vi "测试类型1自动测试一组.vi"() -> ()   [LabVIEW 2010]
uses:
  全局量/试验配置信息.vi
panel:
  in  "测试值":dbl[](array[numeric])
  out "EVENT_KEY":string
  out "bRece":bool
  out "bSend":bool
  out "第几个":i32
  out "bStop":bool
  out "数据组数":i32
  out "第几组":i32
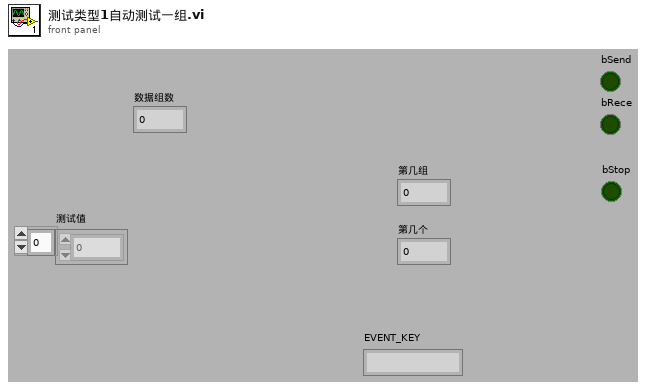
[diagram p1: front panel]
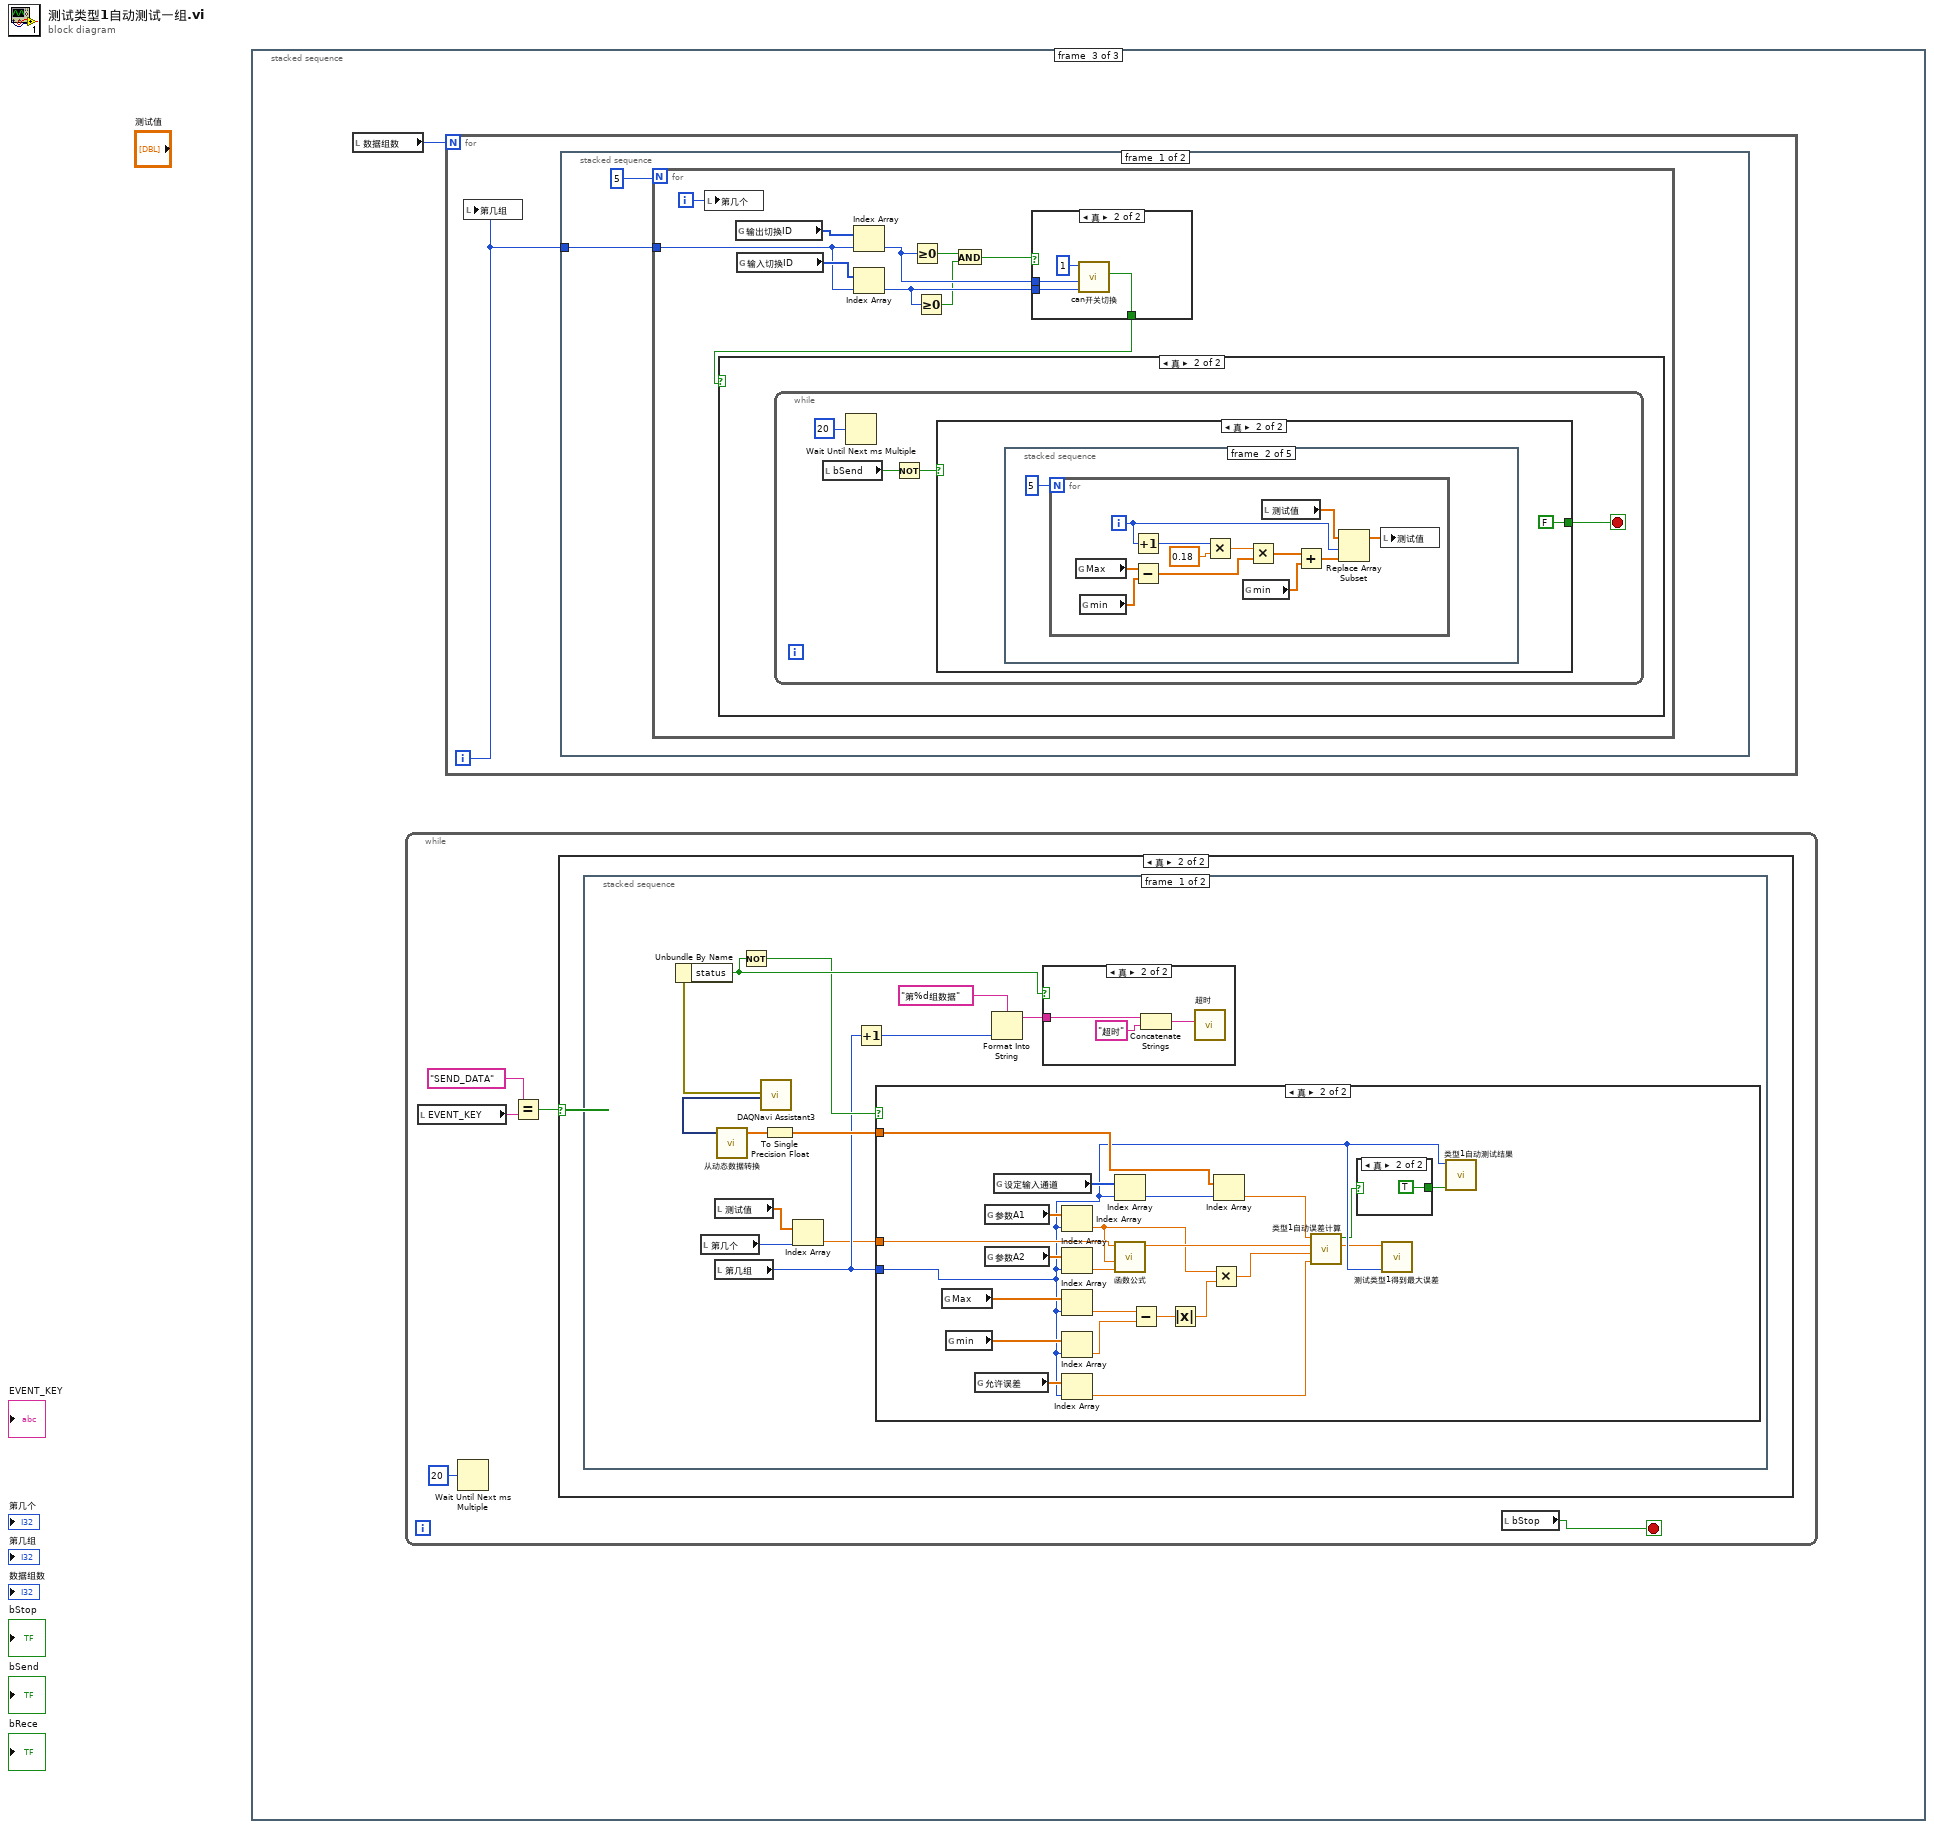
[diagram p0: block diagram]
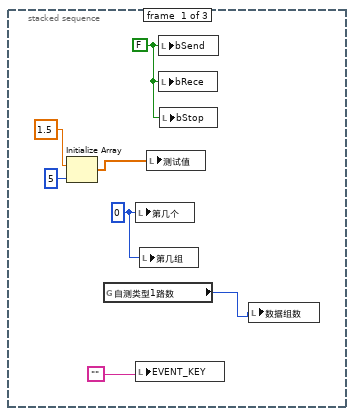
[diagram p2: hidden frame]
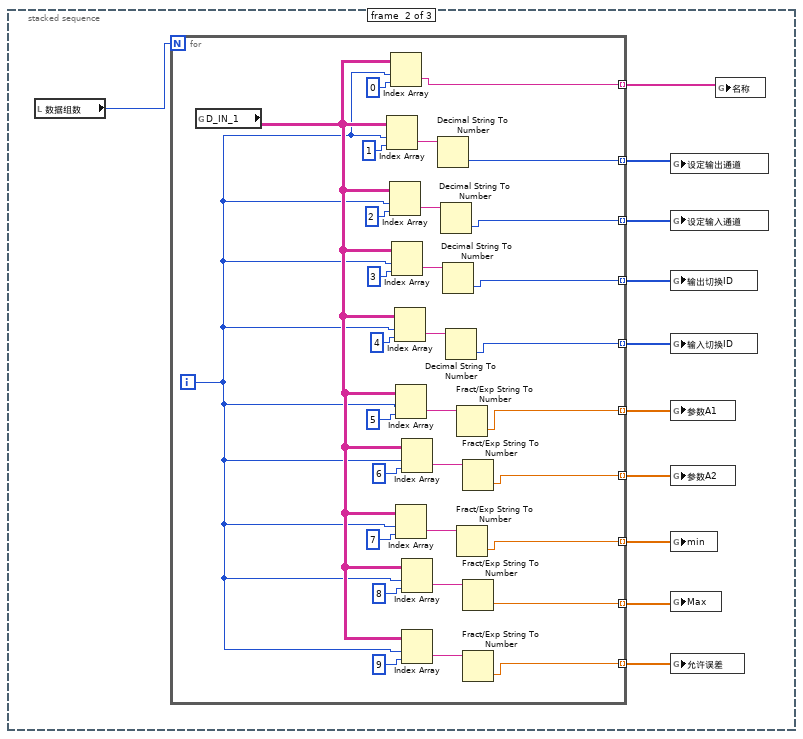
[diagram p3: hidden frame]
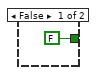
[diagram p7: hidden frame]
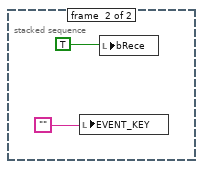
[diagram p8: hidden frame]
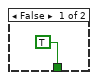
[diagram p9: hidden frame]
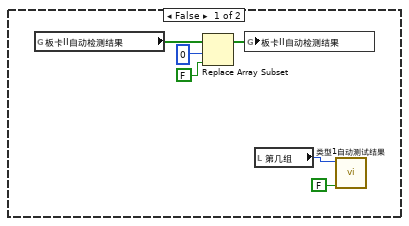
[diagram p10: hidden frame]
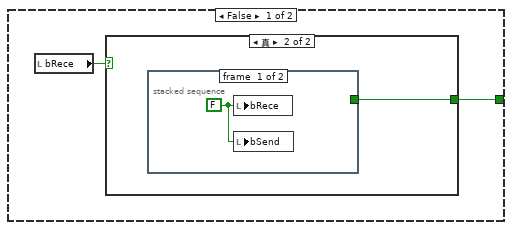
[diagram p11: hidden frame]
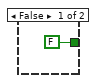
[diagram p12: hidden frame]
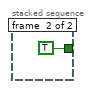
[diagram p13: hidden frame]
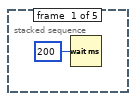
[diagram p14: hidden frame]
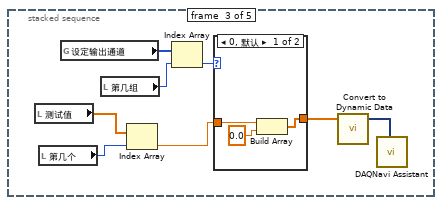
[diagram p15: hidden frame]
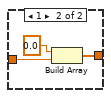
[diagram p16: hidden frame]
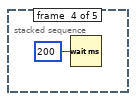
[diagram p17: hidden frame]
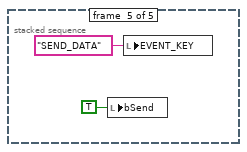
[diagram p18: hidden frame]
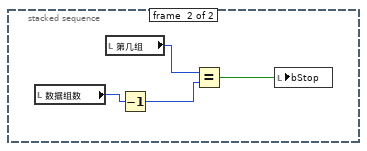
[diagram p19: hidden frame]
diagram:
  n1 = stacked-sequence {
    frame #0 {
      w6 = FALSE
      w7 = 0 ("同步A")
      n2 = Initialize Array(1.5 ("数值"), 5 ("维数大小")) -> (w2:dbl[])
      n3 = global read "试验配置信息.vi" "自测类型1路数"() -> (w1:i32)
      n4 = local write "第几个"(w7) -> ()
      n5 = local write "EVENT_KEY"("") -> ()
      n6 = local write "第几组"(w7) -> ()
      n7 = local write "测试值"(w2) -> ()
      n8 = local write "bSend"(w6) -> ()
      n9 = local write "bRece"(w6) -> ()
      n10 = local write "bStop"(w6) -> ()
      n11 = local write "数据组数"(w1) -> ()
    }
    frame #1 {
      n12 = local read "数据组数"() -> (w9:i32)
      n13 = for {
        N: w9 -> [_]
        tunnel: [w31] -> w10 mode=indexing
        tunnel: [w30] -> w11 mode=indexing
        tunnel: [w29] -> w12 mode=indexing
        tunnel: [w28] -> w13 mode=indexing
        tunnel: [w27] -> w14 mode=indexing
        tunnel: [w26] -> w15 mode=indexing
        tunnel: [w25] -> w16 mode=indexing
        tunnel: [w24] -> w17 mode=indexing
        tunnel: [w23] -> w18 mode=indexing
        tunnel: [w20] -> w8 mode=indexing
        i -> [w19]
        n14 = global read "试验配置信息.vi" "D_IN_1"() -> (w21:string[][])
        n15 = Index Array(array=w21, index (row)=w19, index (col)=1 ("禁用的索引 (列)")) -> (element=w49:string)
        n16 = Index Array(array=w21, index (row)=w19, index (col)=2 ("禁用的索引 (列)")) -> (element=w46:string)
        n17 = Index Array(array=w21, index (row)=w19, index (col)=0 ("禁用的索引 (列)")) -> (element=w20:string)
        n18 = Index Array(array=w21, index (row)=w19, index (col)=3 ("禁用的索引 (列)")) -> (element=w42:string)
        n19 = Index Array(array=w21, index (row)=w19, index (col)=4 ("禁用的索引 (列)")) -> (element=w45:string)
        n20 = Index Array(array=w21, index (row)=w19, index (col)=5 ("禁用的索引 (列)")) -> (element=w40:string)
        n21 = Index Array(array=w21, index (row)=w19, index (col)=7 ("禁用的索引 (列)")) -> (element=w35:string)
        n22 = Index Array(array=w21, index (row)=w19, index (col)=6 ("禁用的索引 (列)")) -> (element=w39:string)
        n23 = Index Array(array=w21, index (row)=w19, index (col)=8 ("禁用的索引 (列)")) -> (element=w36:string)
        n24 = Index Array(array=w21, index (row)=w19, index (col)=9 ("禁用的索引 (列)")) -> (element=w33:string)
        n25 = Decimal String To Number(string=w49) -> (number=w31:i32)  [unwired: 2 in, 1 out]
        n26 = Decimal String To Number(string=w46) -> (number=w30:i32)  [unwired: 2 in, 1 out]
        n27 = Decimal String To Number(string=w42) -> (number=w29:i32)  [unwired: 2 in, 1 out]
        n28 = Decimal String To Number(string=w45) -> (number=w28:i32)  [unwired: 2 in, 1 out]
        n29 = Fract/Exp String To Number(string=w40) -> (number=w27:dbl)  [unwired: 3 in, 1 out]
        n30 = Fract/Exp String To Number(string=w35) -> (number=w25:dbl)  [unwired: 3 in, 1 out]
        n31 = Fract/Exp String To Number(string=w39) -> (number=w26:dbl)  [unwired: 3 in, 1 out]
        n32 = Fract/Exp String To Number(string=w36) -> (number=w24:dbl)  [unwired: 3 in, 1 out]
        n33 = Fract/Exp String To Number(string=w33) -> (number=w23:dbl)  [unwired: 3 in, 1 out]
      }
      n34 = global write "试验配置信息.vi" "设定输出通道"(w10) -> ()
      n35 = global write "试验配置信息.vi" "设定输入通道"(w11) -> ()
      n36 = global write "试验配置信息.vi" "输出切换ID"(w12) -> ()
      n37 = global write "试验配置信息.vi" "输入切换ID"(w13) -> ()
      n38 = global write "试验配置信息.vi" "参数A1"(w14) -> ()
      n39 = global write "试验配置信息.vi" "参数A2"(w15) -> ()
      n40 = global write "试验配置信息.vi" "min"(w16) -> ()
      n41 = global write "试验配置信息.vi" "Max"(w17) -> ()
      n42 = global write "试验配置信息.vi" "允许误差"(w18) -> ()
      n43 = global write "试验配置信息.vi" "名称"(w8) -> ()
    }
    frame #2 {
      n44 = local read "数据组数"() -> (w50:i32)
      n45 = while {
        stop <- w51 stop-if-true
        n46 = local read "EVENT_KEY"() -> (w54:string)
        n47 = Wait Until Next ms Multiple(millisecond multiple=u32 20 ("毫秒倍数")) -> ()  [unwired: 1 out]
        n48 = Equal?(x="SEND_DATA" ("EVENT_KEY"), y=w54) -> (x = y?=w53:bool)
        n49 = case shown="真" w53 {
          frame False {
          }
          frame True {
            n50 = stacked-sequence {
              frame #0 {
                n51 = local read "第几个"() -> (w57:i32)
                n52 = local read "测试值"() -> (w58:dbl[])
                n53 = local read "第几组"() -> (w59:i32)
                n54 = call "DAQNavi Assistant3"() -> ("error out"=w64:errorcluster, "data out(DDT)"=w65:dynamicdata)  [unwired: 2 in, 16 out]
                n55 = Unbundle By Name(w64) -> ("status"=w68:bool)
                n56 = call "从动态数据转换"("Dynamic Data Type"=w65) -> ("Array"=w66:dbl[])  [unwired: 3 in]
                n57 = Not(x=w68) -> (.not. x?=w63:bool)
                n58 = To Single Precision Float(number=w66) -> (single precision float=w67:sgl[])
                n59 = Index Array(array=w58, index=w57) -> (element=w56:dbl)
                n60 = Increment(x=w59) -> (x+1=w62:i32)
                n61 = case shown="真" w63 {
                  tunnel: w67 -> [_ w92]
                  tunnel: w59 -> [_ w81]
                  tunnel: w56 -> [_ w82]
                  frame False {
                  }
                  frame True {
                    n62 = global read "试验配置信息.vi" "Max"() -> (w88:dbl[])
                    n63 = global read "试验配置信息.vi" "min"() -> (w89:dbl[])
                    n64 = global read "试验配置信息.vi" "允许误差"() -> (w87:dbl[])
                    n65 = global read "试验配置信息.vi" "参数A1"() -> (w91:dbl[])
                    n66 = global read "试验配置信息.vi" "参数A2"() -> (w90:dbl[])
                    n67 = global read "试验配置信息.vi" "设定输入通道"() -> (w94:u32[])
                    n68 = Index Array(array=w91, index=w81) -> (element=w74:dbl)
                    n69 = Index Array(array=w90, index=w81) -> (element=w75:dbl)
                    n70 = Index Array(array=w88, index=w81) -> (element=w85:dbl)
                    n71 = Index Array(array=w89, index=w81) -> (element=w84:dbl)
                    n72 = Index Array(array=w87, index=w81) -> (element=w78:dbl)
                    n73 = Index Array(array=w94, index=w81) -> (element=w93:u32)
                    n74 = call "函数公式.vi"("参数 b"=w75, "参数 a"=w74, "设定值 1"=w82) -> ("y"=w79:dbl)  [unwired: 5 in, 1 out]
                    n75 = Subtract(x=w85, y=w84) -> (x-y=w86:dbl)
                    n76 = Absolute Value(x=w86) -> (abs(x)=w73:dbl)
                    n77 = Multiply(x=w74, y=w73) -> (x*y=w72:dbl)
                    n78 = Index Array(array=w92, index=w93) -> (element=w80:sgl)
                    n79 = call "类型1自动误差计算.vi"("允许误差"=w78, "模拟量量程范围"=w72, "设定值_1"=w79, "反馈值_1"=w80) -> ("误差_1"=w77:dbl, "合格_1?"=w76:bool)  [unwired: 5 in, 1 out]
                    n80 = case shown="真" w76 {
                      tunnel: [FALSE TRUE] -> w83
                      frame False {
                      }
                      frame True {
                      }
                    }
                    n81 = call "测试类型1得到最大误差.vi"("第几组"=w81, "新误差值"=w77) -> ()  [unwired: 10 in]
                    n82 = call "类型1自动测试结果.vi"("合格?"=w83, "第几组"=w81) -> ()  [unwired: 10 in]
                  }
                }
                n83 = Format Into String(format string="第%d组数据" ("格式字符串"), w62) -> (resulting string=w61:string)  [unwired: 2 in, 1 out]
                n84 = case shown="真" w68 {
                  tunnel: w61 -> [_ w71]
                  frame False {
                  }
                  frame True {
                    n85 = Concatenate Strings(w71, "超时" ("格式字符串")) -> (w69:string)
                    n86 = call "超时"("Message"=w69) -> ()  [unwired: 9 in, 2 out]
                  }
                }
              }
              frame #1 {
                n87 = local write "EVENT_KEY"("") -> ()
                n88 = local write "bRece"(TRUE) -> ()
              }
            }
          }
        }
        n89 = local read "bStop"() -> (w51:bool)
      }
      n90 = for {
        N: w50 -> [_]
        i -> [w99]
        n91 = local write "第几组"(w99) -> ()
        n92 = stacked-sequence {
          tunnel: w99 -> [w100 _]
          frame #0 {
            n93 = for {
              N: 5 -> [_]
              tunnel: w100 -> [w108]
              i -> [w111]
              n94 = local write "第几个"(w111) -> ()
              n95 = global read "试验配置信息.vi" "输出切换ID"() -> (w110:i32[])
              n96 = global read "试验配置信息.vi" "输入切换ID"() -> (w109:i32[])
              n97 = Index Array(array=w110, index=w108) -> (element=w107:i32)
              n98 = Index Array(array=w109, index=w108) -> (element=w106:i32)
              n99 = Greater Or Equal To 0?(x=w107) -> (x >= 0?=w105:bool)
              n100 = Greater Or Equal To 0?(x=w106) -> (x >= 0?=w104:bool)
              n101 = And(x=w105, y=w104) -> (x .and. y?=w103:bool)
              n102 = case shown="真" w103 {
                tunnel: w107 -> [_ w115]
                tunnel: w106 -> [_ w114]
                tunnel: [TRUE w113] -> w102
                frame False {
                }
                frame True {
                  n103 = call "can开关切换.vi"("输入切换ID"=w114, "输出切换ID"=w115, "函数类型"=1) -> ("成功？"=w113:bool)  [unwired: 7 in]
                }
              }
              n104 = case shown="真" w102 {
                frame False {
                  n105 = global read "试验配置信息.vi" "板卡II自动检测结果"() -> (w122:bool[])
                  n106 = Replace Array Subset(array=w122, new element=FALSE, index=0 ("索引")) -> (w121:bool[])
                  n107 = global write "试验配置信息.vi" "板卡II自动检测结果"(w121) -> ()
                  n108 = local read "第几组"() -> (w117:i32)
                  n109 = call "类型1自动测试结果.vi"("合格?"=FALSE, "第几组"=w117) -> ()  [unwired: 10 in]
                }
                frame True {
                  n110 = while {
                    stop <- w124 stop-if-true
                    n111 = local read "bSend"() -> (w126:bool)
                    n112 = Wait Until Next ms Multiple(millisecond multiple=u32 20 ("毫秒倍数")) -> ()  [unwired: 1 out]
                    n113 = Not(x=w126) -> (.not. x?=w125:bool)
                    n114 = case shown="真" w125 {
                      tunnel: [w127 FALSE] -> w124
                      frame False {
                        n115 = local read "bRece"() -> (w128:bool)
                        n116 = case shown="真" w128 {
                          tunnel: [FALSE w130] -> w127
                          frame False {
                          }
                          frame True {
                            n117 = stacked-sequence {
                              tunnel: [_ TRUE] -> w130
                              frame #0 {
                                w131 = FALSE
                                n118 = local write "bRece"(w131) -> ()
                                n119 = local write "bSend"(w131) -> ()
                              }
                              frame #1 {
                              }
                            }
                          }
                        }
                      }
                      frame True {
                        n120 = stacked-sequence {
                          frame #0 {
                            n121 = Wait (ms)(milliseconds to wait=u32 200 ("等待时间（毫秒）")) -> ()  [unwired: 1 out]
                          }
                          frame #1 {
                            n122 = for {
                              N: 5 -> [_]
                              i -> [w139]
                              n123 = global read "试验配置信息.vi" "Max"() -> (w147:dbl[])
                              n124 = global read "试验配置信息.vi" "min"() -> (w146:dbl[])
                              n125 = Increment(x=w139) -> (x+1=w145:i32)
                              n126 = Subtract(x=w147, y=w146) -> (x-y=w142:dbl[])
                              n127 = Multiply(x=w145, y=0.18) -> (x*y=w143:dbl)
                              n128 = global read "试验配置信息.vi" "min"() -> (w138:dbl[])
                              n129 = Multiply(x=w143, y=w142) -> (x*y=w137:dbl[])
                              n130 = local read "测试值"() -> (w141:dbl[])
                              n131 = Add(x=w137, y=w138) -> (x+y=w136:dbl[])
                              n132 = Replace Array Subset(array=w141, new element=w136, index=w139) -> (w140:dbl[])
                              n133 = local write "测试值"(w140) -> ()
                            }
                          }
                          frame #2 {
                            n134 = local read "测试值"() -> (w150:dbl[])
                            n135 = local read "第几个"() -> (w148:i32)
                            n136 = global read "试验配置信息.vi" "设定输出通道"() -> (w152:u32[])
                            n137 = local read "第几组"() -> (w155:i32)
                            n138 = Index Array(array=w150, index=w148) -> (element=w149:dbl)
                            n139 = Index Array(array=w152, index=w155) -> (element=w153:u32)
                            n140 = case shown="0, 默认" w153 {
                              tunnel: [w158 w161] -> w154
                              tunnel: w149 -> [w156 w159]
                              frame 0, Default {
                                n141 = Build Array(w156, 0.0) -> (w158:dbl[])
                              }
                              frame 1 {
                                n142 = Build Array(0.0, w159) -> (w161:dbl[])
                              }
                            }
                            n143 = call "Convert to Dynamic Data"("Array"=w154) -> ("Dynamic Data Type"=w151:dynamicdata)  [unwired: 3 out]
                            n144 = call "DAQNavi Assistant"("data in(DDT)"=w151) -> ()  [unwired: 2 in, 17 out]
                          }
                          frame #3 {
                            n145 = Wait (ms)(milliseconds to wait=u32 200 ("等待时间（毫秒）")) -> ()  [unwired: 1 out]
                          }
                          frame #4 {
                            n146 = local write "bSend"(TRUE) -> ()
                            n147 = local write "EVENT_KEY"("SEND_DATA" ("EVENT_KEY")) -> ()
                          }
                        }
                      }
                    }
                  }
                }
              }
            }
          }
          frame #1 {
            n148 = local read "数据组数"() -> (w166:i32)
            n149 = local read "第几组"() -> (w168:i32)
            n150 = Decrement(x=w166) -> (x-1=w165:i32)
            n151 = Equal?(x=w168, y=w165) -> (x = y?=w167:bool)
            n152 = local write "bStop"(w167) -> ()
          }
        }
      }
    }
  }
